vi "Set IP Address.vi"(8 "error in (no error)":errorcluster, 10 "IP Address":string="192.168.1.200", 11 "niDTS Comm Telnet in":refnum<class "niDTS Comm Telnet.lvclass">) -> (0 "error out":errorcluster, 3 "niDTS Comm Telnet out":refnum<class "niDTS Comm Telnet.lvclass">)   [LabVIEW 2015, in "niDTS CommLib.lvlib" / "niDTS Comm Telnet.lvclass"]
uses:
  niDTS Comm Telnet.lvclass
  niDTS Comm Telnet.lvclass/niDTS Comm Telnet.ctl
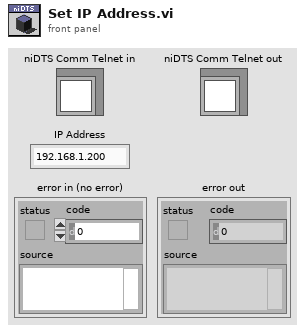
[diagram p1: front panel]
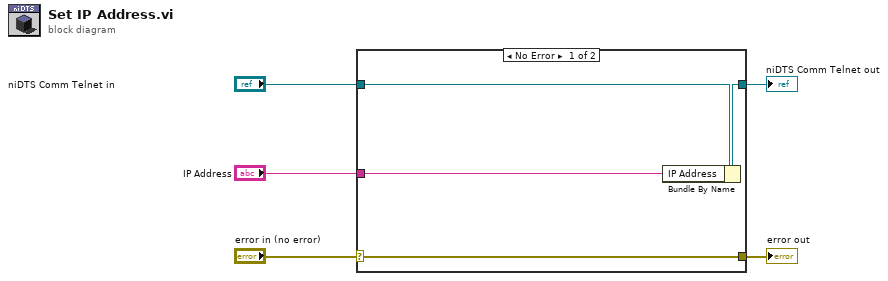
[diagram p0: block diagram]
diagram:
  n1 = case shown="No Error" "error in (no error)" {
    selector: "error in (no error)" -> [w9 w10]
    tunnel: [w9 w10] -> w4
    tunnel: [w7 w11] -> w2
    tunnel: "niDTS Comm Telnet in" -> [w8 w11]
    tunnel: "IP Address" -> [w6 _]
    frame No Error {
      n2 = Bundle By Name(cluster=w8, "IP Address"=w6) -> (w7:refnum<class "niDTS Comm Telnet.lvclass">)
    }
    frame Error {
    }
  }
  "error out" <- w4
  "niDTS Comm Telnet out" <- w2
